vi "MPExxx Error Query (Multiple).vi"(0 "VISA session":refnum<visa-resource-name>, 1 "error in (no error)":errorcluster) -> (2 "dup VISA session":refnum<visa-resource-name>, 3 "error":bool, 4 "error message":string, 5 "error out":errorcluster)   [LabVIEW 2012]
doc: "This VI reads the error queue from the instrument. It expects to see errors in SCPI format (#,\"error message\"). It continues to read from the error queue until it reads a 0, \"No error\"."
panel:
  # "MAGNA-POWER"
  # "Electronics"
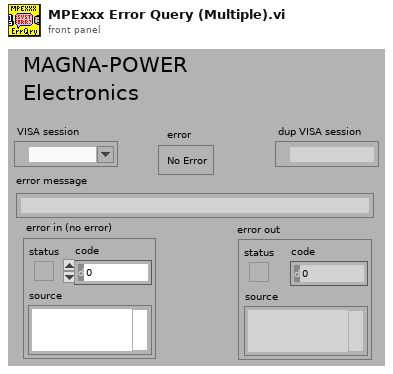
[diagram p1: front panel]
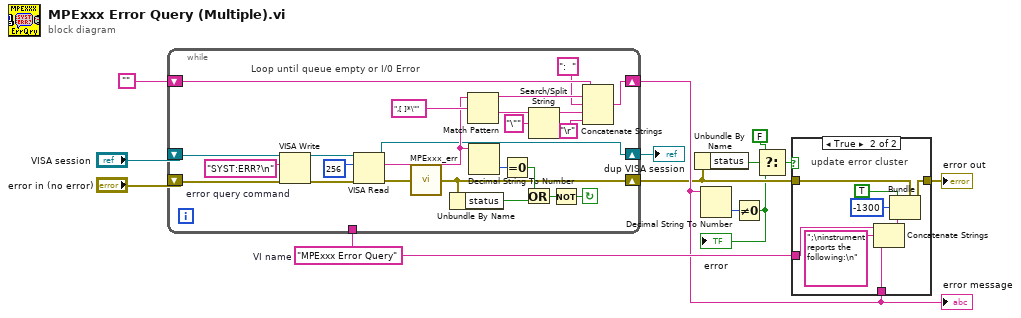
[diagram p0: block diagram]
diagram:
  w12 = "MPExxx Error Query"  # VI name
  n1 = while {
    shift-right: [w20] -> w9
    shift-left: "" -> [w37]
    shift-right: [w14] -> w5
    shift-left: "error in (no error)" -> [w35]
    tunnel: w12 -> [_]
    shift-right: [w21] -> w11
    shift-left: "VISA session" -> [w34]
    stop <- w36 continue-if-true
    w29 = "SYST:ERR?\n"  # error query command
    # "Loop until queue empty or I/0 Error"
    n2 = VISA Write(VISA resource name=w34, write buffer=w29, error in (no error)=w35) -> (VISA resource name out=w28:refnum<visa-resource-name>, error out=w27:errorcluster)  [unwired: 1 out]
    n3 = VISA Read(VISA resource name=w28, byte count=u32 256, error in (no error)=w27) -> (VISA resource name out=w21:refnum<visa-resource-name>, read buffer=w22:string, error out=w15:errorcluster)  [unwired: 1 out]
    n4 = call "MPExxx_err.vi"("error in (no error)"=w15) -> ("error out"=w14:errorcluster)
    n5 = Unbundle By Name(w14) -> ("status"=w31:bool)
    n6 = Match Pattern(string=w22, regular expression=",[ ]*\"") -> (before substring=w25:string, after substring=w23:string)  [unwired: 1 in, 2 out]
    n7 = Decimal String To Number(string=w22) -> (number=w33:i32)  [unwired: 2 in, 1 out]
    n8 = Equal To 0?(x=w33) -> (x = 0?=w32:bool)
    n9 = Or(x=w32, y=w31) -> (x .or. y?=w19:bool)
    n10 = Search/Split String(string=w23, search string/char (-)="\"") -> (substring before match=w17:string)  [unwired: 1 in, 2 out]
    n11 = Not(x=w19) -> (.not. x?=w36:bool)
    n12 = Concatenate Strings(w37, w25, ":  ", w17, "\r") -> (w20:string)
  }
  "error message" <- w9
  "dup VISA session" <- w11
  n13 = Unbundle By Name(w5) -> ("status"=w3:bool)
  n14 = Decimal String To Number(string=w9) -> (number=w10:i32)  [unwired: 2 in, 1 out]
  n15 = Not Equal To 0?(x=w10) -> (x != 0?=w2:bool)
  "error" <- w2
  n16 = Select(t=FALSE, s=w3, f=w2) -> (s? t:f=w1:bool)
  n17 = case shown="True" w1 {
    tunnel: w5 -> [w38 w44]
    tunnel: [w38 w43] -> w8
    tunnel: w9 -> [_ w40]
    tunnel: w12 -> [_ w39]
    frame False {
      # "no instrument errors"
    }
    frame True {
      # "update error cluster"
      n18 = Concatenate Strings(w39, ";\ninstrument reports the following:\n", w40) -> (w42:string)
      n19 = Bundle(cluster=w44, "status"=TRUE, "code"=-1300, "source"=w42) -> (w43:errorcluster)
    }
  }
  "error out" <- w8
